vi "DLTS - reset pulse timing (SubVI).vi"(8 "error in (no error)":errorcluster, 11 "Handle in":T1 {"Handle" format="0x%08x"; "Conn" format="0x%08x"}) -> (0 "error out":errorcluster, 3 "Handle out":T1 {"Handle" format="0x%08x"; "Conn" format="0x%08x"})   [LabVIEW 2019]
doc: "Resets DLTS pulse timing settings after a measurement"
uses:
  <instrlib>/Zurich Instruments LabOne/Public/ziTypeHandle.ctl
  <instrlib>/Zurich Instruments LabOne/Public/Configure/ziSetValueDoubleArray.vi
  <instrlib>/Zurich Instruments LabOne/Zurich Instruments LabOne.lvlib
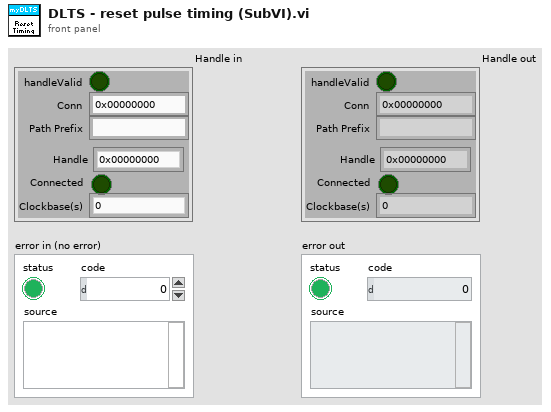
[diagram p1: front panel]
types:
  T1 = typedef "Zurich Instruments LabOne.lvlib/ziTypeHandle.ctl" = cluster{"handleValid":bool, "Conn":u64, "Path Prefix":string, "Handle":u64, "Connected":bool, "Clockbase(s)":dbl}
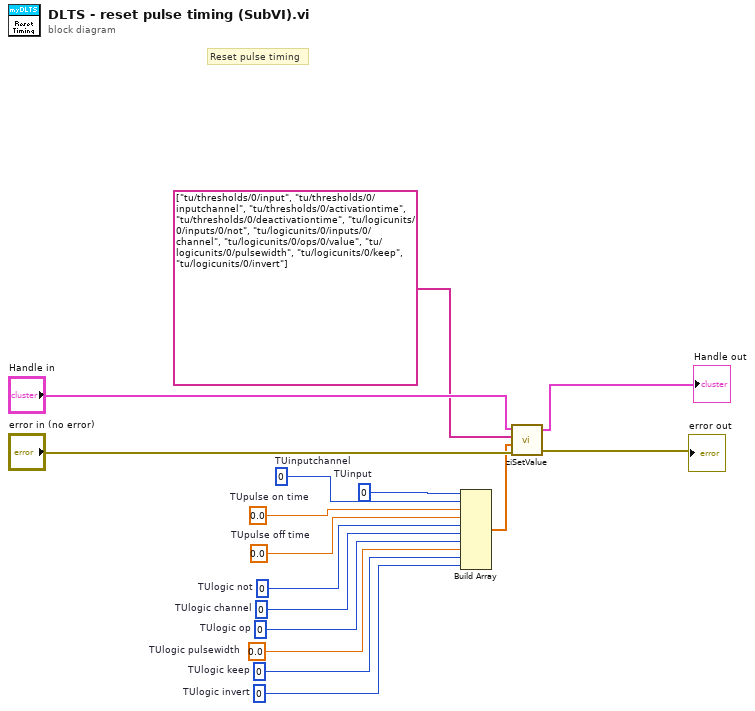
[diagram p0: block diagram]
diagram:
  w12 = 0  # TUlogic invert
  w11 = 0  # TUlogic keep
  w10 = 0.0  # TUlogic pulsewidth
  w9 = 0  # TUlogic op
  w8 = 0  # TUlogic channel
  w7 = 0  # TUlogic not
  w6 = 0  # TUinputchannel
  w5 = 0.0  # TUpulse off time
  w4 = 0.0  # TUpulse on time
  w2 = 0  # TUinput
  # "Reset pulse timing"
  n1 = Build Array(w2, w6, w4, w5, w7, w8, w9, w10, w11, w12) -> (w3:dbl[])
  n2 = call-poly <instrlib>:"ziSetValue.vi"("Error In"="error in (no error)", "Values"=w3, "Paths"=string[] ["tu/thresholds/0/input", "tu/thresholds/0/inputchannel", "tu/thresholds/0/activationtime", "tu/thresholds/0/deactivationtime", "tu/logicunits/0/inputs/0/not", "tu/logicunits/0/inputs/0/channel", "tu/logicunits/0/ops/0/value", "tu/logicunits/0/pulsewidth", "tu/logicunits/0/keep", "tu/logicunits/0/invert"], "Handle In"="Handle in") -> ("Error Out"=→"error out":errorcluster, "Handle Out"=→"Handle out":T1)  [unwired: 1 in]
